vi "Get Cargo Capacity.vi"(8 "error in":errorcluster, 11 "vehicle":refnum<class "Vehicle.lvclass">) -> (0 "error out":errorcluster, 2 "cargo capacity":dbl)   [LabVIEW 2020, in "Vehicle.lvclass"]
doc: "This VI is an example of a dynamic member VI. It returns the cargo capacity for the vehicle."
uses:
  Vehicle.lvclass
  Vehicle.lvclass/Vehicle.ctl
panel:
  # "This VI is an example of a dynamic member VI."
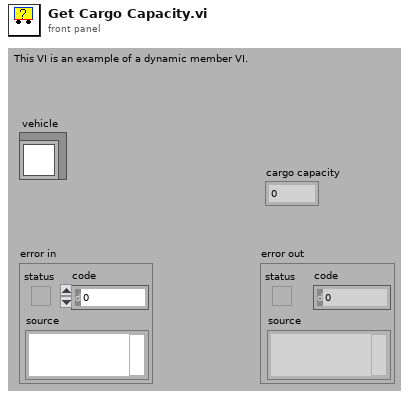
[diagram p1: front panel]
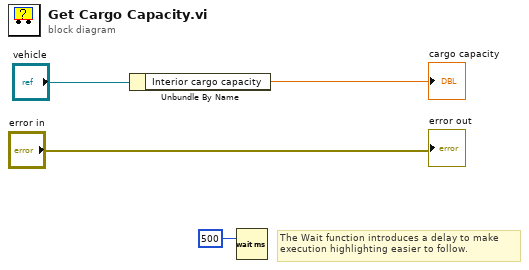
[diagram p0: block diagram]
diagram:
  # "The Wait function introduces a delay to make\nexecution highlighting easier to follow."
  n1 = Unbundle By Name("vehicle") -> ("Interior cargo capacity"=→"cargo capacity":dbl)
  n2 = Wait (ms)(milliseconds to wait=u32 500) -> ()  [unwired: 1 out]
  "error out" <- "error in"
